vi "Add row to database constructor.vi"(8 "error in (no error)":errorcluster, 9 "Ctl Refnum":refnum<vi>, 10 "Self Enqueuer":refnum<class "Message Enqueuer.lvclass">, 11 "Add Row to Database in":refnum<class "Add Row to Database.lvclass">) -> (0 "error out":errorcluster, 3 "Add Row to Database out":refnum<class "Add Row to Database.lvclass">)   [LabVIEW 2020, in "Panel Form Controller.lvlib" / "Add Row to Database.lvclass"]
uses:
  Add Row to Database.lvclass
  C:/Users/User/Desktop/Raman Program/LV-Database-OOP/source/Database OOP/Button Libraries/Button/Button Class/Button.lvclass
  <vilib>/ActorFramework/Message Enqueuer/Message Enqueuer.lvclass
  Database OOP/Button Libraries/Button/Button Class/Button.lvclass/Button.ctl
  Add Row to Database.lvclass/Add Row to Database.ctl
  Database OOP/Button Libraries/Button/Button Class/Button.lvclass
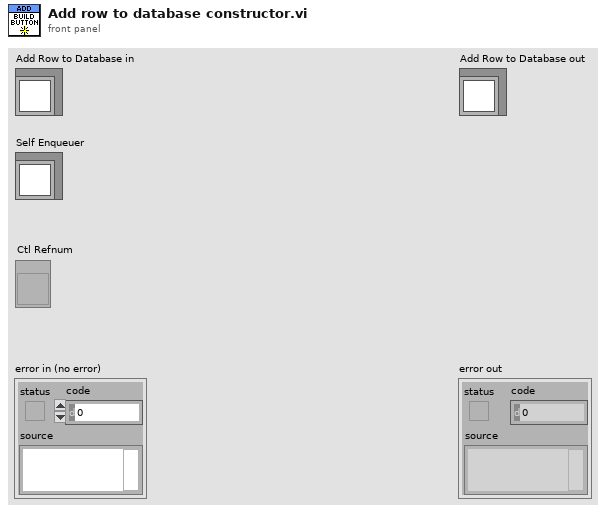
[diagram p1: front panel]
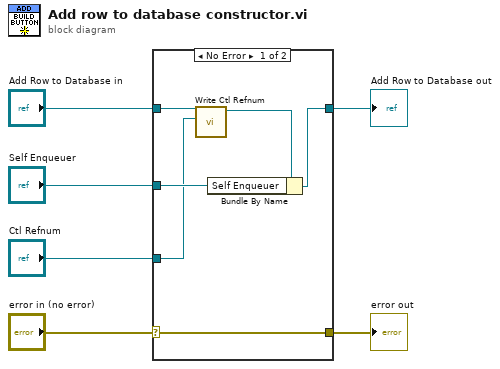
[diagram p0: block diagram]
diagram:
  n1 = case shown="No Error" "error in (no error)" {
    selector: "error in (no error)" -> [w12 w14]
    tunnel: [w12 w14] -> w5
    tunnel: [w9 w13] -> w3
    tunnel: "Add Row to Database in" -> [w11 w13]
    tunnel: "Self Enqueuer" -> [w8 _]
    tunnel: "Ctl Refnum" -> [w7 _]
    frame No Error {
      n2 = call "Write Ctl Refnum.vi"("Ctl Refnum"=w7, "Button in"=w11) -> ("Button out"=w10:refnum<class "Add Row to Database.lvclass">)  [unwired: 8 in, 1 out]
      n3 = Bundle By Name(cluster=w10, "Self Enqueuer"=w8) -> (w9:refnum<class "Add Row to Database.lvclass">)
    }
    frame Error {
    }
  }
  "error out" <- w5
  "Add Row to Database out" <- w3
